vi "Root Element.vi"(8 "error in (no error)":errorcluster, 11 "Config Manager in":refnum<class "Config Manager.lvclass">) -> (0 "error out":errorcluster, 2 "Root Element":refnum<class "Config Element.lvclass">, 3 "Config Manager out":refnum<class "Config Manager.lvclass">)   [LabVIEW 2023, in "CDM-Config.lvlib" / "Config Manager.lvclass"]
doc: "Returns the root element of the config. The root of all configs is an unnamed, usually valueless, element to serve as the top-level parent for any names elements with no \"parent\". (All elements that have a single string value element in their hierarchy name array)."
uses:
  Config Manager.lvclass
  Config Element/Config Element.lvclass
  Config Manager.lvclass/Config Manager.ctl
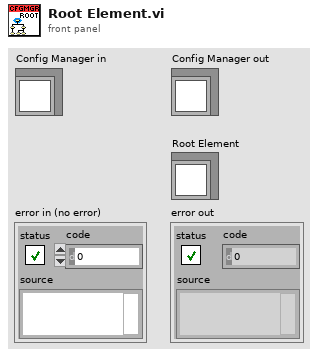
[diagram p1: front panel]
types:
  T1 = typedef "CDM-Config.lvlib/Config Manager.lvclass/Ref Data.ctl" = cluster{"Elements":refnum<class "Config Element.lvclass">[], "Hierarchy Map":map{string[], i32}, "Element Map":map{refnum<class "Config Element.lvclass">, i32}}
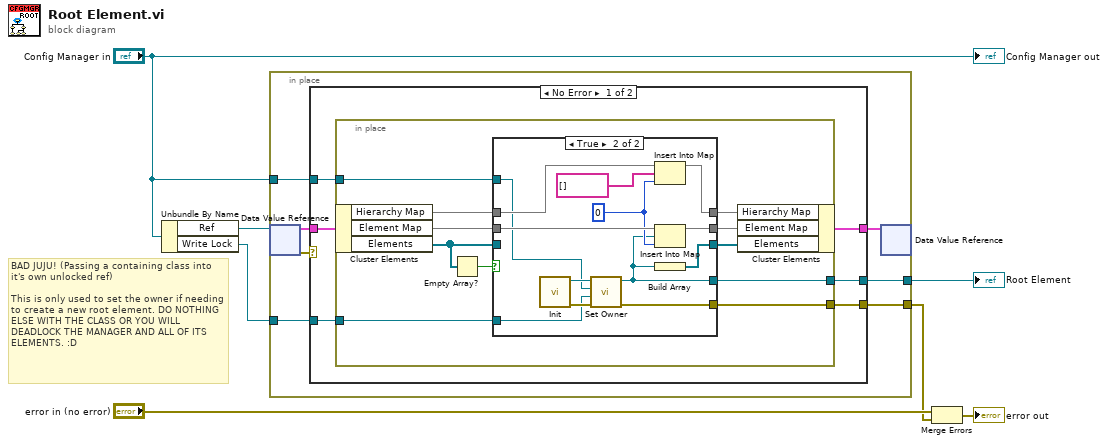
[diagram p0: block diagram]
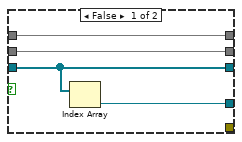
[diagram p2: hidden frame]
diagram:
  # "BAD JUJU! (Passing a containing class into it's own unlocked ref)\n\nThis is only used to set the owner if needing to create a new root element. DO NOTHING ELSE WITH THE CLASS OR YOU WILL DEADLOCK THE MANAGER AND ALL OF ITS ELEMENTS. :D"
  n1 = Unbundle By Name("Config Manager in") -> ("Ref"=w7:refnum<data-value>, "Write Lock"=w3:refnum<notifier>)
  n2 = in-place {
    in-place-border: [w12] -> w2
    in-place-border: [w10] -> w4
    in-place-border: w3 -> [w9]
    in-place-border: "Config Manager in" -> [w8]
    n3 = in-place-dvr #1(w7) -> (w14:T1, w11:errorcluster)
    n4 = case shown="No Error" w11 {
      selector: w11 -> [_ w49]
      tunnel: w14 -> [w20 w50]
      tunnel: [w19 w50] -> w13
      tunnel: [w18 _] -> w12
      tunnel: [w17 w49] -> w10
      tunnel: w9 -> [w16 _]
      tunnel: w8 -> [w15 _]
      frame No Error {
        n5 = in-place {
          in-place-border: [w29] -> w18
          in-place-border: [w24] -> w17
          in-place-border: w16 -> [w22]
          in-place-border: w15 -> [w21]
          n6 = in-place-cluster #2(w20) -> ("Hierarchy Map"=w27:map{string[], i32}, "Element Map"=w28:map{refnum<class "Config Element.lvclass">, i32}, "Elements"=w31:refnum<class "Config Element.lvclass">[])
          n7 = Empty Array?(array=w31) -> (empty?=w23:bool)
          n8 = case shown="True" w23 {
            tunnel: w31 -> [w35 _]
            tunnel: [w35 w48] -> w30
            tunnel: [w34 w39] -> w29
            tunnel: w28 -> [w33 w44]
            tunnel: w27 -> [w32 w47]
            tunnel: [w33 w43] -> w26
            tunnel: [w32 w45] -> w25
            tunnel: [_ w38] -> w24
            tunnel: w22 -> [_ w37]
            tunnel: w21 -> [_ w36]
            frame False {
              n9 = Index Array(array=w35) -> (element=w34:refnum<class "Config Element.lvclass">)  [unwired: 1 in]
            }
            frame True {
              w42 = 0 ("value")
              n10 = call "Init.vi"() -> ("error out"=w40:errorcluster, "Config Element out"=w41:refnum<class "Config Element.lvclass">)  [unwired: 10 in]
              n11 = call "Set Owner.vi"("error in (no error)"=w40, "Write Lock"=w37, "Owner"=w36, "Config Element in"=w41) -> ("error out"=w38:errorcluster, "Config Element out"=w39:refnum<class "Config Element.lvclass">)  [unwired: 6 in]
              n12 = Insert Into Map(map in=w47, key=string[] [], value=w42) -> (map out=w45:map{string[], i32})  [unwired: 2 out]
              n13 = Insert Into Map(map in=w44, key=w39, value=w42) -> (map out=w43:map{refnum<class "Config Element.lvclass">, i32})  [unwired: 2 out]
              n14 = Build Array(w39) -> (w48:refnum<class "Config Element.lvclass">[])
            }
          }
          n15 = in-place-cluster #2("Hierarchy Map"=w25, "Element Map"=w26, "Elements"=w30) -> (w19:T1)
        }
      }
      frame Error {
      }
    }
    n16 = in-place-dvr #1(w13) -> ()  [unwired: 2 out]
  }
  "Root Element" <- w2
  n17 = Merge Errors("error in (no error)", w4) -> (→"error out":errorcluster)
  "Config Manager out" <- "Config Manager in"
